vi "Finalize.vi"(7 "Actor in":refnum<class "Actor.lvclass">, 8 "Error in":errorcluster, 10 "Msg Output":refnum<class "Msg Output.lvclass">) -> (0 "Error out":errorcluster, 5 "Actor out":refnum<class "Actor.lvclass">)   [LabVIEW 2020, in "jettl.lvlib"]
uses:
  jettl.lvlib
  Msg Output/Msg Output.lvclass
  Actor/Actor.lvclass
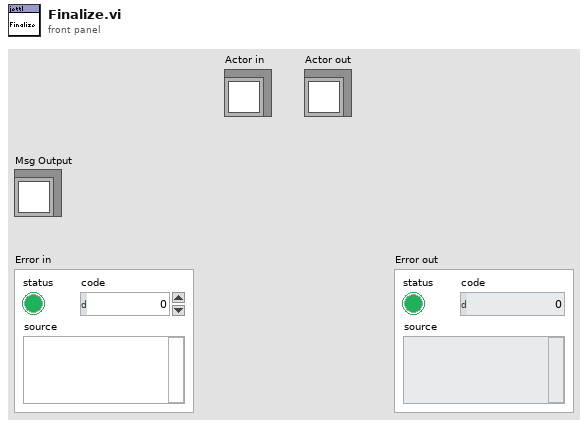
[diagram p1: front panel]
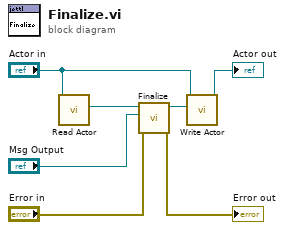
[diagram p0: block diagram]
diagram:
  n1 = call-dynamic "Read Actor.vi"("Actor in"="Actor in") -> ("Actor"=w5:refnum<class "Actor.lvclass">)  [unwired: 10 in]
  n2 = call-dynamic "Finalize.vi"("Error in"="Error in", "Msg Output"="Msg Output", "Actor in"=w5) -> ("Error out"=→"Error out":errorcluster, "Actor out"=w4:refnum<class "Actor.lvclass">)  [unwired: 7 in]
  n3 = call-dynamic "Write Actor.vi"("Actor"=w4, "Actor in"="Actor in") -> ("Actor out"=→"Actor out":refnum<class "Actor.lvclass">)  [unwired: 9 in]
